vi "Generate Tabs.vi"(8 "error in (no error)":errorcluster, 10 "indent":i32) -> (0 "error out":errorcluster, 2 "Tabs":string)   [LabVIEW 2017, in "Advanced Variant Tools.lvlib"]
doc: "Generates n number of tabs, where n is determined by the current Pretty Print Level."
uses:
  Advanced Variant Tools.lvlib
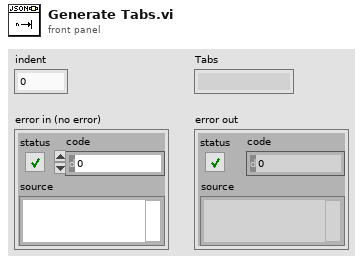
[diagram p1: front panel]
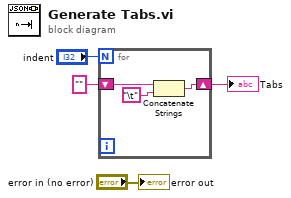
[diagram p0: block diagram]
diagram:
  n1 = for {
    N: "indent" -> [_]
    shift-right: [w5] -> w3
    shift-left: "" -> [w7]
    n2 = Concatenate Strings(w7, "\t") -> (w5:string)
  }
  "Tabs" <- w3
  "error out" <- "error in (no error)"
